vi "Method 2 Ultrasonic.vi"   [LabVIEW 2012]
uses:
  <vilib>/NXT/Subs/MotorOutput.ctl
types:
  T1 = typedef "MotorOutput.ctl" = u8
  T2 = typedef "LVHSConnector.ctl" = refnum<class "BrickReference.lvclass">
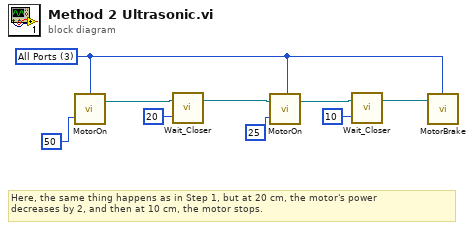
[diagram p0: block diagram]
diagram:
  w7 = T1 3 items=["Port A"=0, "Port B"=1, "Port C"=2, "Ports A & B"=4, "Ports A & C"=5, "Ports B & C"=6, "All Ports"=3] ("Output Port (All Ports)")
  # "Here, the same thing happens as in Step 1, but at 20 cm, the motor's power\ndecreases by 2, and then at 10 cm, the motor stops."
  n1 = call <vilib>:"MotorOn.vi"("Power (75)"=50, "Output Port (All Ports)"=w7) -> ("NXT/EV3"=w6:T2)  [unwired: 2 in]
  n2 = call <vilib>:"Wait_Closer.vi"("Distance (40)"=i16 20, "NXT/EV3"=w6) -> ("NXT/EV3"=w5:T2)  [unwired: 2 in]
  n3 = call <vilib>:"MotorOn.vi"("Power (75)"=25, "NXT/EV3"=w5, "Output Port (All Ports)"=w7) -> ("NXT/EV3"=w4:T2)  [unwired: 1 in]
  n4 = call <vilib>:"Wait_Closer.vi"("Distance (40)"=i16 10, "NXT/EV3"=w4) -> ("NXT/EV3"=w3:T2)  [unwired: 2 in]
  n5 = call <vilib>:"MotorBrake.vi"("NXT/EV3"=w3, "Port (All Ports)"=w7) -> ()  [unwired: 2 in, 1 out]
